vi "GlobalVariables.vi"() -> ()   [LabVIEW 2019]
panel:
  out "HistogramEnabled":bool
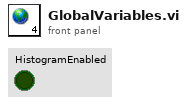
[diagram p1: front panel]
diagram:
